vi "clearAllFromRun.vi"(8 "error in (no error)":errorcluster, 10 "Listbox in":refnum<vi>, 11 "ExperimentRunner in":refnum<class "ExperimentRunner.lvclass">) -> (0 "error out":errorcluster, 2 "Listbox out":refnum<vi>, 3 "ExperimentRunner out":refnum<class "ExperimentRunner.lvclass">)   [LabVIEW 2009, in "Views.lvlib" / "ExperimentControl.lvlib" / "ExperimentRunner.lvclass"]
uses:
  ExperimentRunner.lvclass
  ExperimentRunner.lvclass/ExperimentRunner.ctl
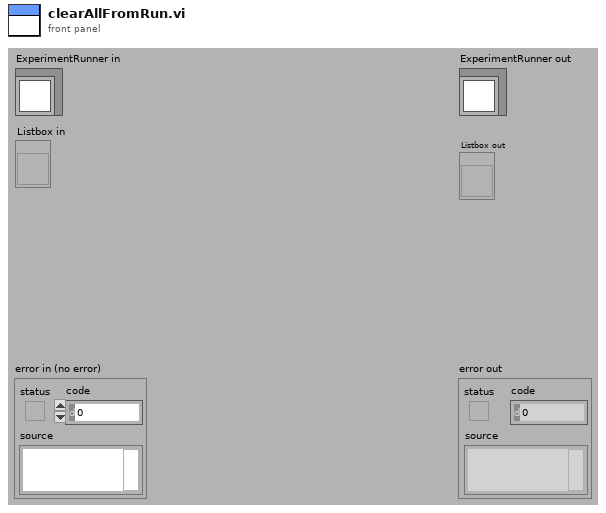
[diagram p1: front panel]
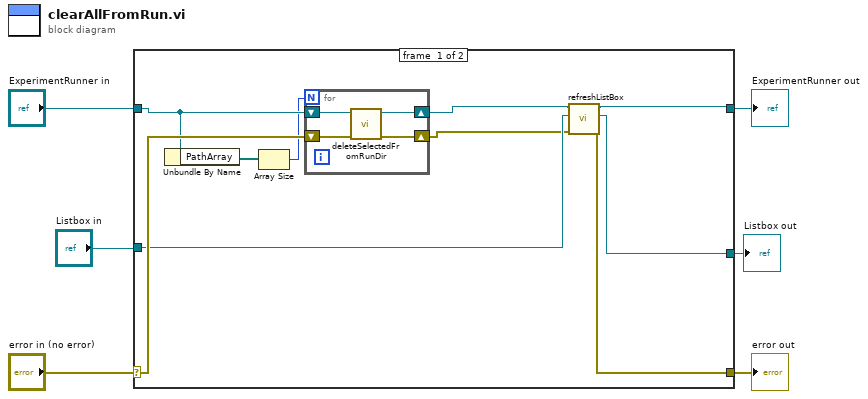
[diagram p0: block diagram]
diagram:
  n1 = case shown="No Error" "error in (no error)" {
    selector: "error in (no error)" -> [w16 w22]
    tunnel: [w7 w22] -> w5
    tunnel: [w11 w21] -> w3
    tunnel: "ExperimentRunner in" -> [w15 w21]
    tunnel: "Listbox in" -> [w10 _]
    tunnel: [w9 _] -> w1
    frame #0 {
      n2 = Unbundle By Name(w15) -> ("PathArray"=w14:path[])
      n3 = Array Size(array=w14) -> (size(s)=w13:i32)
      n4 = for {
        N: w13 -> [_]
        shift-right: [w19] -> w12
        shift-left: w15 -> [w20]
        shift-right: [w17] -> w8
        shift-left: w16 -> [w18]
        n5 = call "deleteSelectedFromRunDir.vi"("error in (no error)"=w18, "ExperimentRunner in"=w20) -> ("error out"=w17:errorcluster, "ExperimentRunner out"=w19:refnum<class "ExperimentRunner.lvclass">)  [unwired: 8 in]
      }
      n6 = call "refreshListBox.vi"("error in (no error)"=w8, "Listbox"=w10, "ExperimentRunner in"=w12) -> ("error out"=w7:errorcluster, "Listbox out"=w9:refnum<vi>, "ExperimentRunner out"=w11:refnum<class "ExperimentRunner.lvclass">)  [unwired: 6 in]
    }
    frame #1 {
    }
  }
  "error out" <- w5
  "ExperimentRunner out" <- w3
  "Listbox out" <- w1
